vi "clearpath_manage_incoming.vi"(1 "Message Data Cluster In":T1, 2 "Data Queue":refnum<queue>, 3 "Xmit Queue":refnum<queue>) -> (0 "Message Data Cluster Out":T1)   [LabVIEW 2011, in "clearpath_interface.lvlib"]
doc: "Manage message data buffer, processing CCP messages which have been fully received. New data messages are placed into the Data Queue, and acknowledgements to commands/data requests are marked by removing their message types from the Ack List."
uses:
  clearpath_interface.lvlib
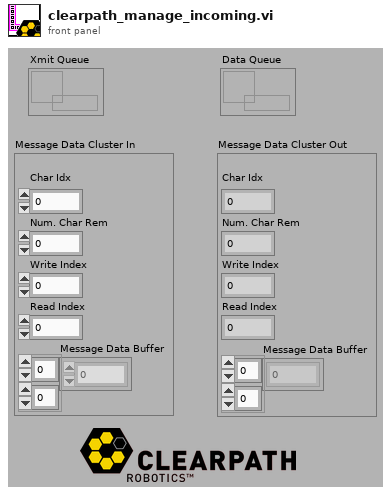
[diagram p1: front panel]
types:
  T1 = cluster{"\nChar Idx":u8, "Num. Char Rem":u8, "Write Index":u8, "Read Index":u8, "Message Data Buffer":u8[][]}
  T2 = cluster{"Message Data Buffer":u8[], "Message Length":u16, "Message Type":u16}
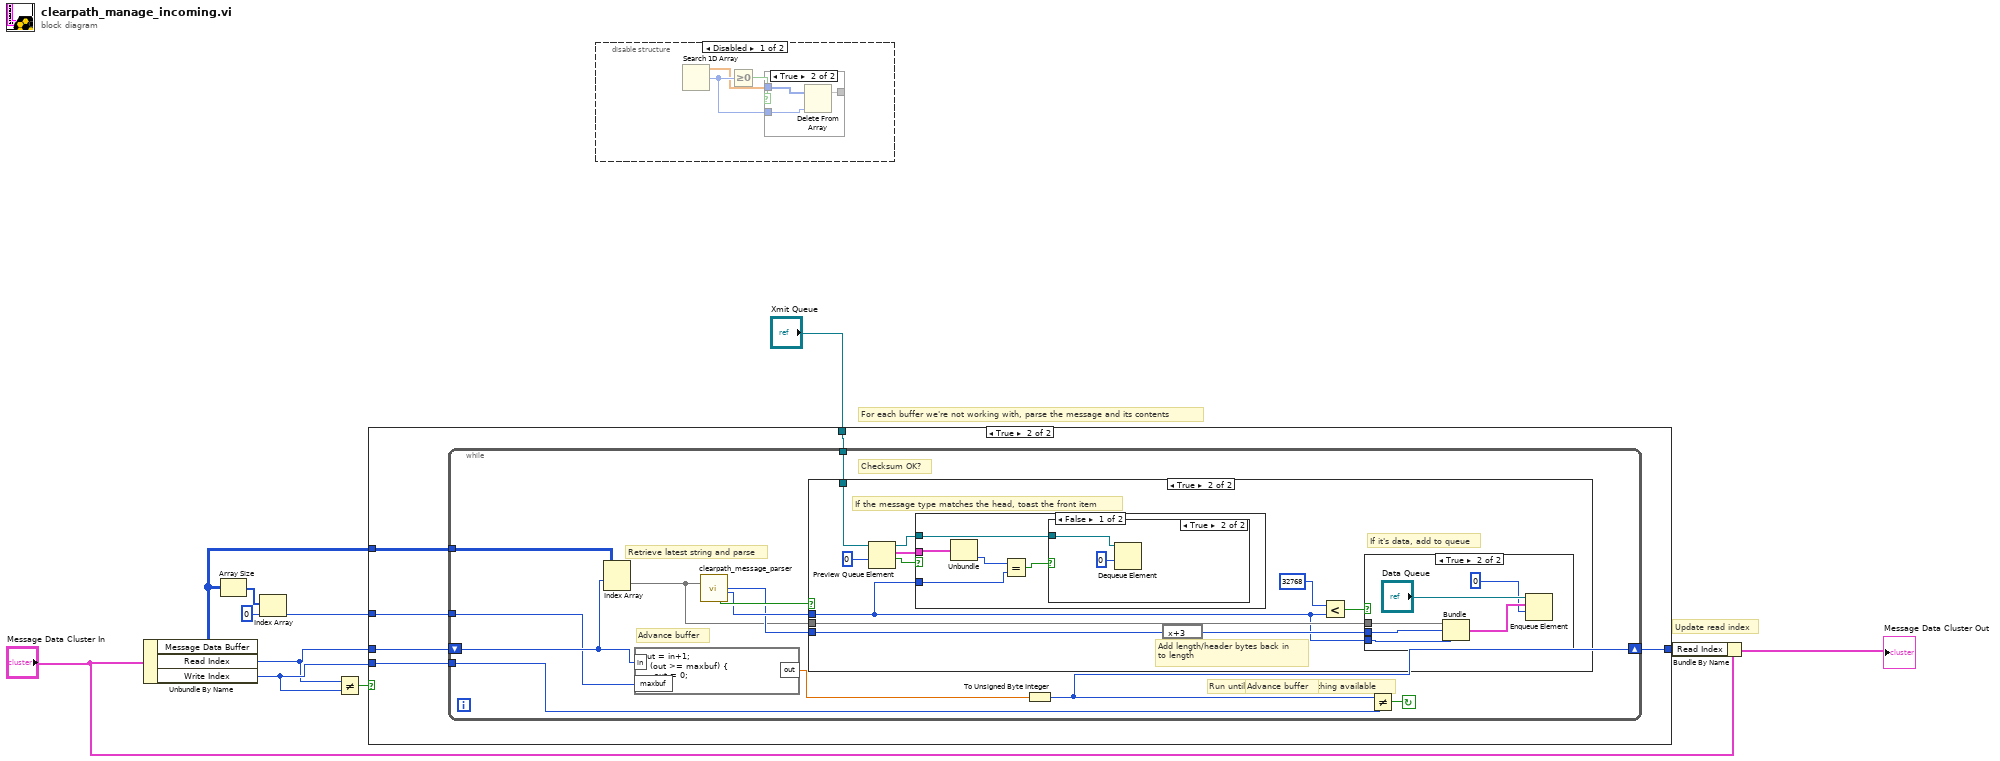
[diagram p0: block diagram]
diagram:
  # "Update read index"
  # "For each buffer we're not working with, parse the message and its contents"
  n1 = Unbundle By Name("Message Data Cluster In") -> ("Message Data Buffer"=w3:u8[][], "Read Index"=w9:u8, "Write Index"=w10:u8)
  n2 = Array Size(array=w3) -> (size(s)=w4:i32[])
  n3 = Index Array(array=w4, index=0) -> (element=w2:i32)
  n4 = Not Equal?(x=w9, y=w10) -> (x != y?=w6:bool)
  n5 = case shown="True" w6 {
    tunnel: w9 -> [w12 w17]
    tunnel: w3 -> [_ w18]
    tunnel: [w12 w16] -> w7
    tunnel: w10 -> [_ w15]
    tunnel: w2 -> [_ w14]
    tunnel: "Xmit Queue" -> [_ w13]
    frame False {
    }
    frame True {
      n6 = while {
        tunnel: w18 -> [w25]
        shift-right: [w24] -> w16
        shift-left: w17 -> [w30]
        tunnel: w15 -> [w23]
        tunnel: w14 -> [w22]
        tunnel: w13 -> [w19]
        stop <- w29 continue-if-true
        # "Run until we're read everything available"
        # "Advance buffer"
        # "Retrieve latest string and parse"
        # "Checksum OK?"
        # "Advance buffer"
        n7 = Index Array(array=w25, index (row)=w30) -> (element=w20:u8[])  [unwired: 1 in]
        n8 = formula code="out = in+1;\nif (out >= maxbuf) {\n    out = 0;\n}"("in"=w30, "maxbuf"=w22) -> ("out"=w28:dbl)
        n9 = call "clearpath_message_parser.vi"("Input Array"=w20) -> ("Message Length"=w21:u16, "Message Type"=w26:u16, "Checksum Valid"=w27:bool)  [unwired: 1 in, 2 out]
        n10 = case shown="True" w27 {
          tunnel: w26 -> [_ w32]
          tunnel: w21 -> [_ w41]
          tunnel: w20 -> [_ w38]
          tunnel: w19 -> [_ w34]
          frame False {
          }
          frame True {
            # "Add length/header bytes back in\nto length"
            # "If it's data, add to queue"
            # "If the message type matches the head, toast the front item"
            n11 = Preview Queue Element(queue=w34, timeout in ms (-1)=0) -> (queue out=w31:refnum<queue>, element=w36:cluster{i32[], i32, i32}, timed out?=w33:bool)  [unwired: 1 in, 1 out]
            n12 = case shown="False" w33 {
              tunnel: w36 -> [w46 _]
              tunnel: w32 -> [w44 _]
              tunnel: w31 -> [w43 _]
              frame False {
                n13 = Unbundle(w46) -> (w45:i32)  [unwired: 2 out]
                n14 = Equal?(x=w45, y=w44) -> (x = y?=w42:bool)
                n15 = case shown="True" w42 {
                  tunnel: w43 -> [_ w48]
                  frame False {
                  }
                  frame True {
                    n16 = Dequeue Element(queue=w48, timeout in ms (-1)=0) -> ()  [unwired: 1 in, 4 out]
                  }
                }
              }
              frame True {
              }
            }
            n17 = expression code="x+3"(w41) -> (w37:u16)
            n18 = Less?(x=u16 32768 ("y"), y=w32) -> (x < y?=w40:bool)
            n19 = case shown="True" w40 {
              tunnel: w38 -> [_ w54]
              tunnel: w37 -> [_ w53]
              tunnel: w32 -> [_ w52]
              frame False {
              }
              frame True {
                n20 = Bundle("Message Data Buffer"=w54, "Message Length"=w53, "Message Type"=w52) -> (w50:T2)  [unwired: 1 in]
                n21 = Enqueue Element(queue="Data Queue", element=w50, timeout in ms (-1)=0) -> ()  [unwired: 1 in, 3 out]
              }
            }
          }
        }
        n22 = To Unsigned Byte Integer(number=w28) -> (unsigned 8bit integer=w24:u8)
        n23 = Not Equal?(x=w24, y=w23) -> (x != y?=w29:bool)
      }
    }
  }
  n24 = disable-structure shown="Disabled" {
    frame Disabled {
      n25 = Search 1D Array() -> (1D array=w57:dbl[], element=w55:dbl, index of element=w58:i32)  [unwired: 1 in]
      n26 = Greater Or Equal To 0?(x=w58) -> (x >= 0?=w59:bool)
      n27 = case shown="True" w59 {
        tunnel: w58 -> [_ w63]
        tunnel: w57 -> [w60 w62]
        tunnel: [w60 w61] -> w56
        frame False {
        }
        frame True {
          n28 = Delete From Array(array=w62, index=w63) -> (array with subset deleted=w61)  [unwired: 1 in, 1 out]
        }
      }
    }
    frame Enabled {
    }
  }
  n29 = Bundle By Name(cluster="Message Data Cluster In", "Read Index"=w7) -> (→"Message Data Cluster Out":T1)
